vi "FlpLib AlphaBetaToDQ_noSine 0.vi"(0 "alpha":sgl format="%#_32g", 1 "cosx":sgl, 2 "sinx":sgl, 5 "beta":sgl format="%#_32g") -> (4 "direct":sgl, 6 "quadrature":sgl)   [LabVIEW 2017]
uses:
  <userlib>/_NI FLP Library/FPGA/outsideSCTL/FlpLib Multiply Shared Instance 0.vi
  <userlib>/_NI FLP Library/FPGA/outsideSCTL/FlpLib Subtract Shared Instance 0.vi
  <userlib>/_NI FLP Library/FPGA/outsideSCTL/FlpLib Add Shared Instance 0.vi
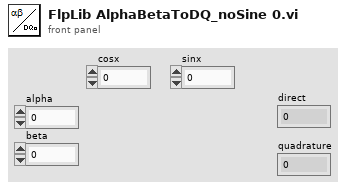
[diagram p1: front panel]
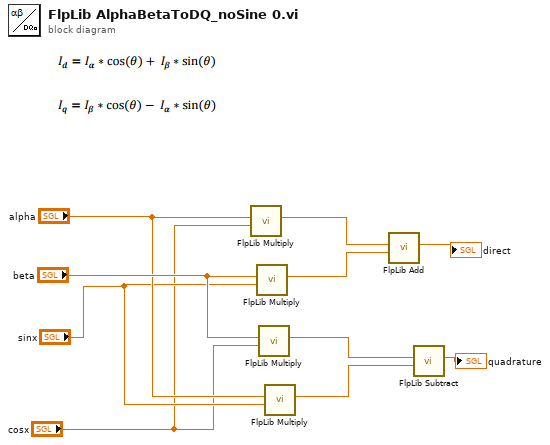
[diagram p0: block diagram]
diagram:
  n1 = call-poly <userlib>:"FlpLib Multiply.vi"("y"="cosx", "x"="alpha") -> ("x*y"=w5:sgl)  [unwired: 5 in]
  n2 = call-poly <userlib>:"FlpLib Multiply.vi"("y"="sinx", "x"="beta") -> ("x*y"=w4:sgl)  [unwired: 5 in]
  n3 = call-poly <userlib>:"FlpLib Multiply.vi"("y"="cosx", "x"="beta") -> ("x*y"=w3:sgl)  [unwired: 5 in]
  n4 = call-poly <userlib>:"FlpLib Multiply.vi"("y"="sinx", "x"="alpha") -> ("x*y"=w2:sgl)  [unwired: 5 in]
  n5 = call-poly <userlib>:"FlpLib Add.vi"("y"=w4, "x"=w5) -> ("x+y"=→"direct":sgl)  [unwired: 5 in]
  n6 = call-poly <userlib>:"FlpLib Subtract.vi"("y"=w2, "x"=w3) -> ("x-y"=→"quadrature":sgl)  [unwired: 5 in]
